vi "Main.vi"() -> ()   [LabVIEW 2014]
doc: "You can create an arbitrarily complex hierarchy of widgets. For example, you can put a Multiple Document Interface (MDI) inside a splitter inside a tab inside a... (and so on). This ability lets you compose almost any GUI arrangement that you can think of.\n\nWhat's more, you can do all this at run-time, and your widgets can auto-resize themselves in layouts.\n\n\nCopyright (c) 2019 Sze Howe Koh.\nThis code is licensed under the MIT license."
uses:
  Widget Builders/Tab Widget Builder/Tab Widget Builder.lvclass
  Global Chart List Action.ctl
  <vilib>/addons/LQ/Qt Widgets/QWidget/setVisible.vi
  <vilib>/addons/LQ/LQ Core/LQCoreEngine/LQCoreEngine.lvclass
  Widgets/Growable Widget/Growable Widget.lvclass
panel:
  in  "Stop Button":bool
  # "Prerequisite knowledge/experience\n- Example 6. Reusing Components Dynamically from the \"Hello World - Introduction to Widgets\" series\n\n- Dynamic dispatching for LabVIEW classes\n   http://zone.ni.com/reference/en-XX/help/371361M-01/lvconcepts/creating_classes/#Dynamic_Dispatch\n\n- Functional Globals or Action Engines\n   http://forums.ni.com/t5/LabVIEW/Community-Nugget-4-08-2007-Action-Engines/td-p/503801\n\n\nDescription\nYou can create an arbitrarily complex hierarchy of widgets. For example, you can put a Multiple Document\nInterface (MDI) inside a splitter inside a tab inside a... (and so on). This ability lets you compose almost any\nGUI arrangement that you can think of.\n\nWhat's more, you can do all this at run-time, and your widgets can auto-resize themselves in layouts.\n\n\nInstructions\n1. Run this VI\n2. Select \"Button Gallery\"  from the drop-down menu\n3. Enter a label of your choice in the \"New widget label\" field\n4. Click \"Add Widget\"\n5. Repeat steps #2 - #4, selecting different widgets from the drop-down menu\n\n\nShowcase\n- Dynamically composing a GUI, based on user input\n- The virtually unlimited ways to nest widgets\n- Dynamically resizing layouts\n- A variety of widgets (including MDI)\n\n\nKnown Issues\n- If you select \"Tab Widget\", \"Tool Box\", \"Horizontal Splitter\", \"Vertical Splitter, or \"MDI Area\", LabVIEW will\n   freeze when you transition from Run mode back to Edit mode (i.e. when you stop this VI).\n    - This is caused by an issue inside LabVIEW; NI is tracking this issue under CAR #690115."
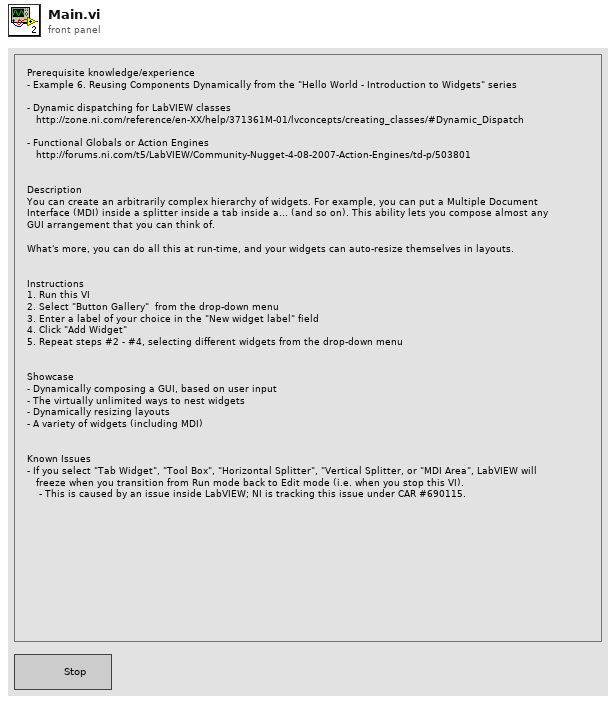
[diagram p1: front panel]
types:
  T1 = typedef "Global Chart List Action.ctl" = enum16{"Clear", "Register Chart", "Append to Charts"}
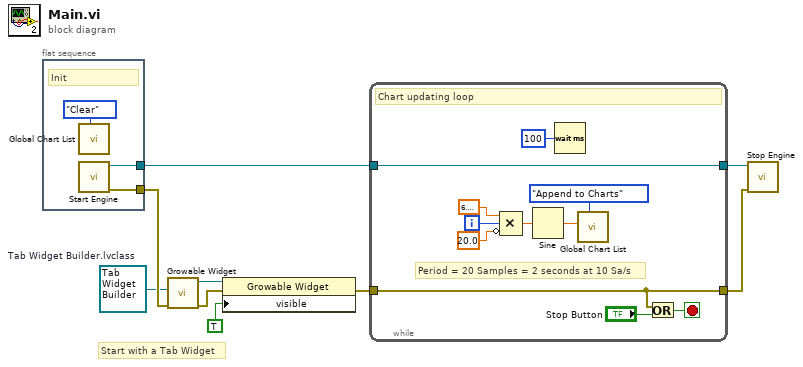
[diagram p0: block diagram]
diagram:
  w1 = refnum<class "Tab Widget Builder.lvclass"> refnum  # Tab Widget Builder.lvclass
  # "Start with a Tab Widget"
  n1 = flat-sequence {
    tunnel: [w12] -> w8
    tunnel: [w11] -> w7
    frame #0 {
      # "Init"
      n2 = call "Global Chart List.vi"("Action"=Global_Chart_List_Action."Clear") -> ()  [unwired: 11 in]
      n3 = call <vilib>:"Start Engine.vi"() -> ("Error Out"=w11:errorcluster, "New Engine"=w12:refnum<class "LQCoreEngine.lvclass">)  [unwired: 10 in]
    }
  }
  n4 = call "Growable Widget.vi"("Error In"=w7, "Widget Builder"=w1) -> ("Error Out"=w5:errorcluster, "New Growable Widget"=w6:refnum<class "Growable Widget.lvclass">)  [unwired: 8 in]
  n5 = property class="Growable Widget"(reference=w6, error in=w5, "visible"=TRUE) -> (error out=w3:errorcluster)  [unwired: 1 out]
  n6 = while {
    tunnel: w3 -> [w14]
    tunnel: [w14] -> w2
    tunnel: w8 -> [w22]
    tunnel: [w22] -> w9
    i -> [w20]
    stop <- w15 stop-if-true
    # "Period = 20 Samples = 2 seconds at 10 Sa/s"
    # "Chart updating loop"
    n7 = Compound Arithmetic op=MULTIPLY(6.283185307179586, w20, invert 20.0 ("value")) -> (w17:dbl)
    n8 = Sine(x=w17) -> (sin(x)=w16:dbl)
    n9 = Wait (ms)(milliseconds to wait=u32 100) -> ()  [unwired: 1 out]
    n10 = call "Global Chart List.vi"("Action"=Global_Chart_List_Action."Append to Charts", "Value"=w16) -> ()  [unwired: 10 in]
    n11 = Or(x=w14, y="Stop Button") -> (x .or. y?=w15:bool)
  }
  n12 = call <vilib>:"Stop Engine.vi"("Error In"=w2, "LQCoreEngine"=w9) -> ()  [unwired: 9 in, 1 out]
